vi "fill.vi"(8 "error in (no error)":errorcluster, 11 "afRed in":refnum<class "afRed.lvclass">) -> (0 "error out":errorcluster, 3 "afRed out":refnum<class "afRed.lvclass">)   [LabVIEW 2017, in "afRed.lvclass"]
uses:
  afRed.lvclass
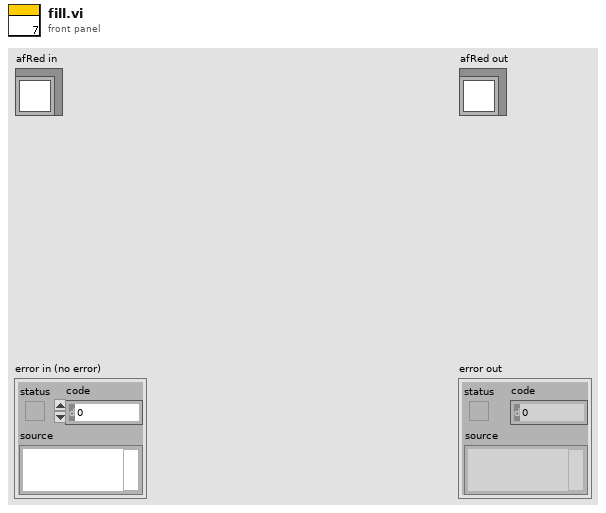
[diagram p1: front panel]
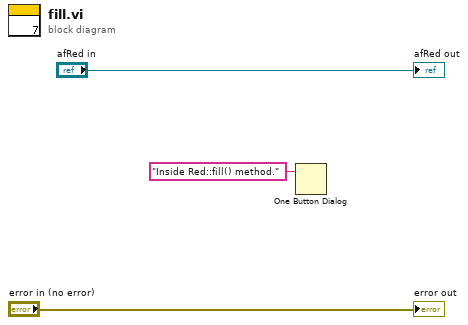
[diagram p0: block diagram]
diagram:
  n1 = One Button Dialog(message="Inside Red::fill() method.") -> ()  [unwired: 1 in, 1 out]
  "error out" <- "error in (no error)"
  "afRed out" <- "afRed in"
